vi "一键清洗流程.vi"(10 "项名":string[](array[string]), 11 "参数下拉列表":u16(ring) items=["总磷"=1, "总氮"=2]) -> ()   [LabVIEW 2016, in "斯坦道总氮.lvlib"]
uses:
  <vilib>/Plasmionique/MB Master/MB_Master/MB_Master.lvclass
panel:
  out "数组":i32[](array[numeric])
  out "枚举":T1(ring)
  out "数值":i32
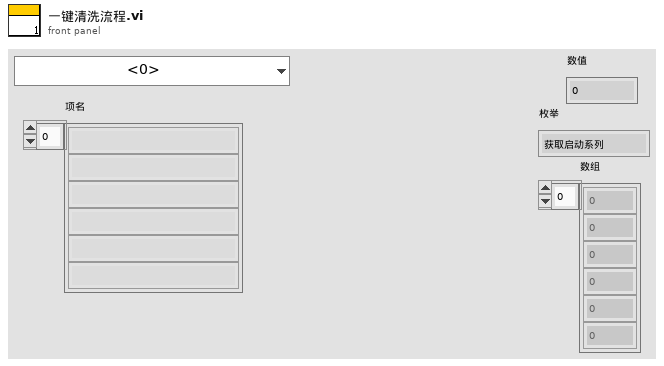
[diagram p1: front panel]
types:
  T1 = enum16{"获取启动系列", "获取启动项", "启动", "测试中", "单个流程测试结束", "判断是否结束", "结束"}
  T2 = cluster{"系统时间":timestamp, "工作状态":u16, "测量模式":enum16{"待机", "连续模式", "周期模式", "定点模式", "受控模式", "手动模式"}, "告警代码":u16, "故障代码":u16, "日志代码":u16, "软件版本":u16, "F0":sgl, "F1":sgl, "F2":sgl, "F3":sgl, "T":sgl, "H":sgl, "id":u16, "flowid":u16, "量程":u16, "总磷控温温度1":sgl, "营养盐控温温度2":sgl, "ADC":sgl}
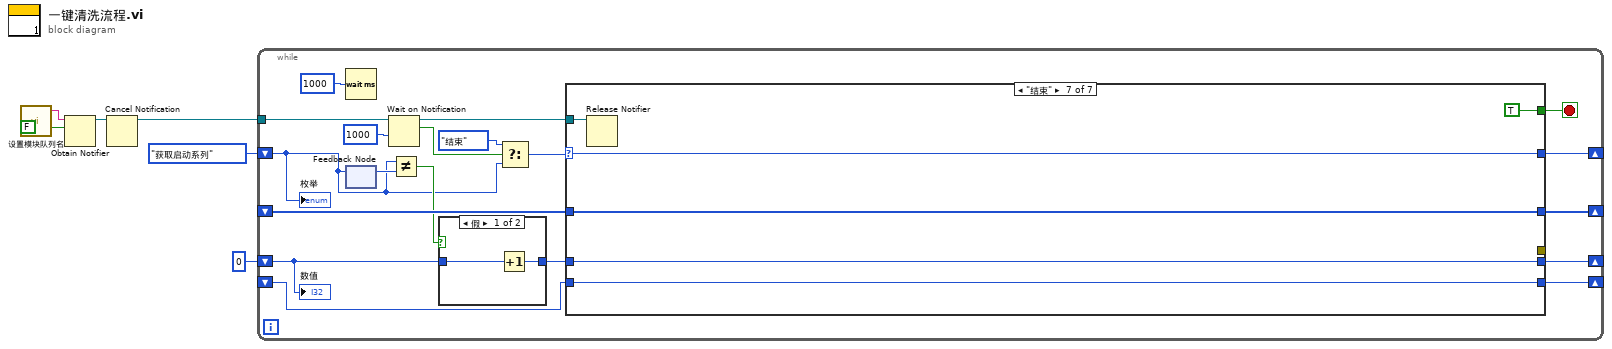
[diagram p0: block diagram]
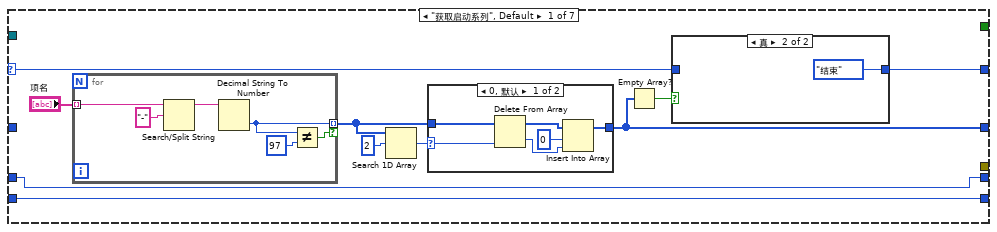
[diagram p3: hidden frame]
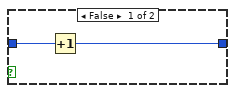
[diagram p5: hidden frame]
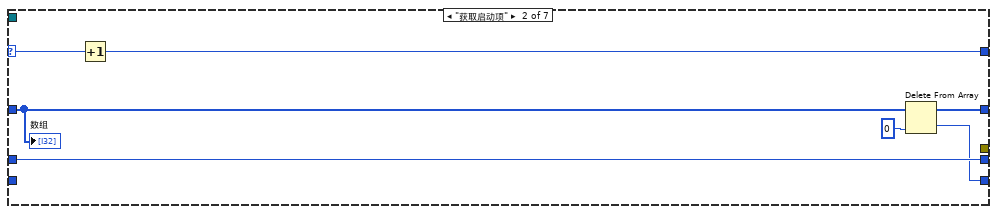
[diagram p6: hidden frame]
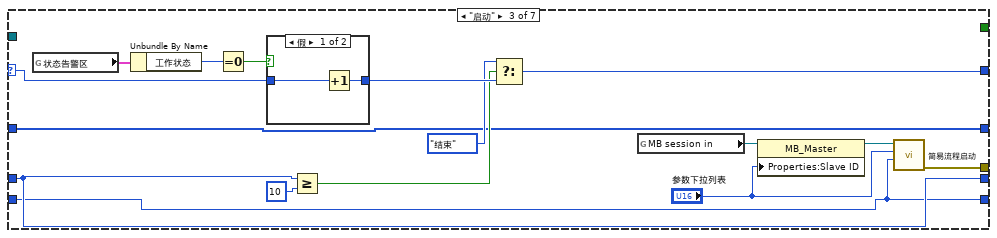
[diagram p7: hidden frame]
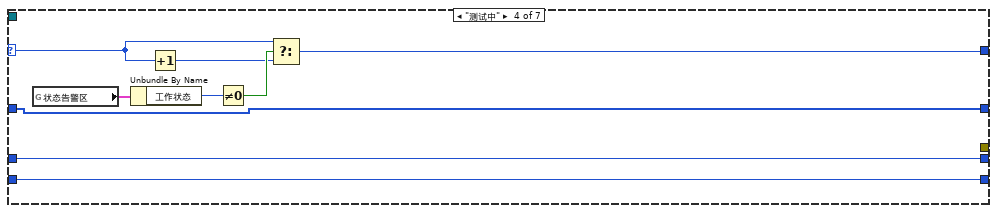
[diagram p9: hidden frame]
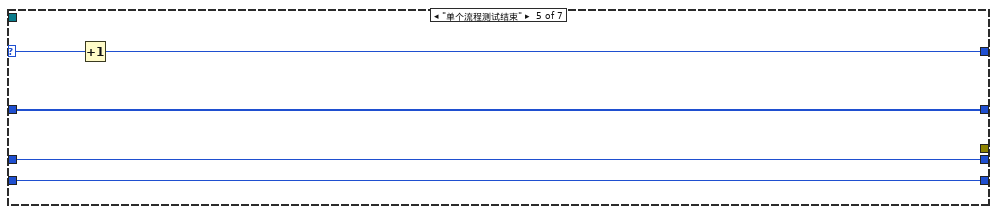
[diagram p10: hidden frame]
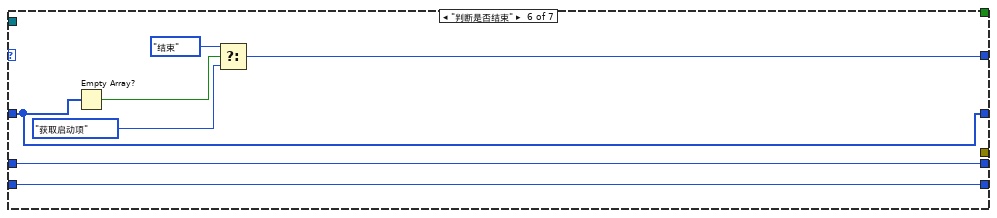
[diagram p11: hidden frame]
diagram:
  n1 = call "设置模块队列名.vi"() -> ("Msg"=w3:string)  [unwired: 5 in]
  n2 = Obtain Notifier(name (unnamed)=w3, notification data type=FALSE) -> (notifier out=w2:refnum<notifier>)  [unwired: 2 in, 2 out]
  n3 = Cancel Notification(0:w2) -> (8:w1:refnum<notifier>)  [unwired: 1 in, 2 out]
  n4 = while {
    shift-right: [w23] -> _
    shift-left: T1."获取启动系列" ("枚举") -> [w10]
    shift-right: [w25] -> _
    shift-left: _ -> [w24]
    shift-right: [w18] -> _
    shift-left: 0 -> [w20]
    shift-right: [w15] -> _
    shift-left: _ -> [w14]
    tunnel: w1 -> [w13]
    stop <- w17 stop-if-true
    n5 = Wait (ms)(milliseconds to wait=u32 1000 ("等待时间（毫秒）")) -> ()  [unwired: 1 out]
    n6 = feedback #1() -> (w22:T1)  [unwired: 1 in]
    n7 = feedback-in #1(w10) -> ()
    n8 = Wait on Notification(notifier=w13, timeout in ms (-1)=1000 ("超时毫秒(-1)")) -> (notifier out=w7:refnum<notifier>, notification=w11:bool)  [unwired: 2 in, 2 out]
    n9 = Not Equal?(x=w10, y=w22) -> (x != y?=w21:bool)
    n10 = case shown="假" w21 {
      tunnel: w20 -> [w27 _]
      tunnel: [w26 _] -> w19
      frame False {
        n11 = Increment(x=w27) -> (x+1=w26:i32)
      }
      frame True {
      }
    }
    n12 = Select(t=T1."结束", s=w11, f=w10) -> (s? t:f=w9:T1)
    n13 = case shown="\"结束\"" w9 {
      selector: w9 -> [w36 w60 w73 w84 w92 _ w105]
      tunnel: [w31 w56 w62 w81 w91 w99 w104] -> w25
      tunnel: w24 -> [_ w57 w62 w81 w91 w99 w104]
      tunnel: [w35 w59 w65 w85 w90 w97 w105] -> w23
      tunnel: [_ _ w69 _ _ _ _] -> _
      tunnel: w19 -> [w34 w58 w68 w82 w93 w100 w106]
      tunnel: [w34 w58 w68 w82 w93 w100 w106] -> w18
      tunnel: [_ _ _ _ _ _ TRUE] -> w17
      tunnel: [w29 w54 w61 w80 w89 w95 w102] -> w15
      tunnel: w14 -> [w29 _ w61 w80 w89 w95 w102]
      tunnel: w7 -> [_ _ _ _ _ _ w101]
      frame "获取启动系列", Default {
        n14 = for {
          tunnel: "项名" -> [w51] mode=indexing
          tunnel: [w50] -> w32 mode=indexing if=w48
          n15 = Search/Split String(string=w51, search string/char (-)="-" ("搜索字符串/字符(-)")) -> (substring before match=w52:string)  [unwired: 1 in, 2 out]
          n16 = Decimal String To Number(string=w52) -> (number=w50:i32)  [unwired: 2 in, 1 out]
          n17 = Not Equal?(x=w50, y=97) -> (x != y?=w48:bool)
        }
        n18 = Search 1D Array(1D array=w32, element=2 ("元素")) -> (index of element=w28:i32)  [unwired: 1 in]
        n19 = case shown="0, 默认" w28 {
          selector: w28 -> [w38 _]
          tunnel: w32 -> [w43 w44]
          tunnel: [w39 w44] -> w31
          frame 0, Default {
            n20 = Delete From Array(array=w43, index=w38) -> (deleted portion=w42:i32, array with subset deleted=w41:i32[])  [unwired: 1 in]
            n21 = Insert Into Array(array=w41, index=0 ("索引"), new element=w42) -> (w39:i32[])
          }
          frame -1 {
          }
        }
        n22 = Empty Array?(array=w31) -> (empty?=w30:bool)
        n23 = case shown="真" w30 {
          tunnel: w36 -> [w46 _]
          tunnel: [w45 T1."结束" ("枚举")] -> w35
          frame False {
            n24 = Increment(x=w46) -> (x+1=w45:T1)
          }
          frame True {
          }
        }
      }
      frame "获取启动项" {
        n25 = Increment(x=w60) -> (x+1=w59:T1)
        n26 = Delete From Array(array=w57, index=0 ("长度")) -> (deleted portion=w54:i32, array with subset deleted=w56:i32[])  [unwired: 1 in]
        "数组" <- w57
      }
      frame "启动" {
        n27 = global read "VAR总磷总氮全局变量.vi" "状态告警区"() -> (w71:T2)
        n28 = Unbundle By Name(w71) -> ("工作状态"=w70:u16)
        n29 = Equal To 0?(x=w70) -> (x = 0?=w66:bool)
        n30 = case shown="假" w66 {
          tunnel: w73 -> [w78 w79]
          tunnel: [w77 w79] -> w72
          frame False {
            n31 = Increment(x=w78) -> (x+1=w77:T1)
          }
          frame True {
          }
        }
        n32 = Greater Or Equal?(x=w68, y=10) -> (x >= y?=w64:bool)
        n33 = Select(t=T1."结束" ("枚举"), s=w64, f=w72) -> (s? t:f=w65:T1)
        n34 = global read "VAR总磷总氮全局变量.vi" "MB session in"() -> (w74:refnum<class "MB_Master.lvclass">)
        n35 = property class="MB_Master"(reference=w74, "Properties:Slave ID"="参数下拉列表") -> (reference out=w76:refnum<class "MB_Master.lvclass">)  [unwired: 1 in, 1 out]
        n36 = call "简易流程启动.vi"("简易流程"=w61, "参数Id"="参数下拉列表", "MB session in"=w76) -> ("error out"=w69:errorcluster)  [unwired: 7 in, 1 out]
      }
      frame "测试中" {
        n37 = global read "VAR总磷总氮全局变量.vi" "状态告警区"() -> (w88:T2)
        n38 = Unbundle By Name(w88) -> ("工作状态"=w87:u16)
        n39 = Increment(x=w84) -> (x+1=w83:T1)
        n40 = Not Equal To 0?(x=w87) -> (x != 0?=w86:bool)
        n41 = Select(t=w84, s=w86, f=w83) -> (s? t:f=w85:T1)
      }
      frame "单个流程测试结束" {
        n42 = Increment(x=w92) -> (x+1=w90:T1)
      }
      frame "判断是否结束" {
        n43 = Empty Array?(array=w99) -> (empty?=w98:bool)
        n44 = Select(t=T1."结束" ("枚举"), s=w98, f=T1."获取启动项") -> (s? t:f=w97:T1)
      }
      frame "结束" {
        n45 = Release Notifier(notifier=w101) -> ()  [unwired: 2 in, 3 out]
      }
    }
    "数值" <- w20
    "枚举" <- w10
  }
